vi "Subgroup Spectrum Lines.vi"(0 "spectra":T2(array[cluster]), 9 "system info in":refnum<class "EP System Info.lvclass">, 11 "error in (no error)":errorcluster) -> (4 "harmonic subgroups complex spectra":cluster{"f0":dbl, "df":dbl, "vectors":cdb[]}[](array[cluster]), 6 "interharmonic subgroups complex spectra":cluster{"f0":dbl, "df":dbl, "vectors":cdb[]}[](array[cluster]), 10 "system info out":refnum<class "EP System Info.lvclass">, 15 "error out":errorcluster)   [LabVIEW 2014, in "NI_EP_Power Quality.lvlib"]
doc: "Performs subgrouping of 10/12-cycle step spectra to harmonic and interharmonic spectra according to IEC 61000-4-7:2009. Use the Complex To Polar function to convert the results of this VI to magnitude and phase spectra. Use the Complex To Re/Im function to convert the results of this VI to real and imaginary spectra.\n\nThis VI supports measuring single-line and multiple-line systems."
uses:
  <vilib>/addons/Electrical Power/PQ/NI_EP_Power Quality.lvlib
  <vilib>/addons/Electrical Power/PQ/Common/Controls/ep_AI Data Channel.ctl
  <vilib>/addons/Electrical Power/PQ/Common/Classes/System Info/EP System Info.lvclass
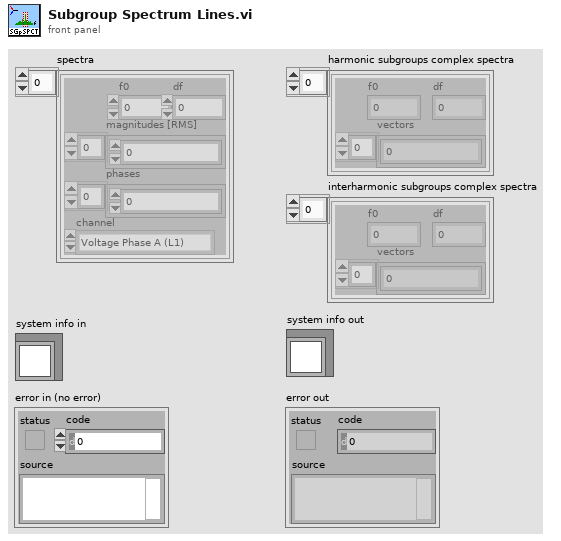
[diagram p1: front panel]
types:
  T1 = typedef "NI_EP_Power Quality.lvlib/ep_AI Data Channel.ctl" = enum16{"Voltage Phase A (L1)", "Voltage Phase B (L2)", "Voltage Phase C (L3)", "Voltage Phase N (Neutral)", "Current Phase A (L1)", "Current Phase B (L2)", "Current Phase C (L3)", "Current Phase N (Neutral)"}
  T2 = cluster{"f0":dbl, "df":dbl, "magnitudes [RMS]":dbl[], "phases":dbl[], "channel":T1}[]
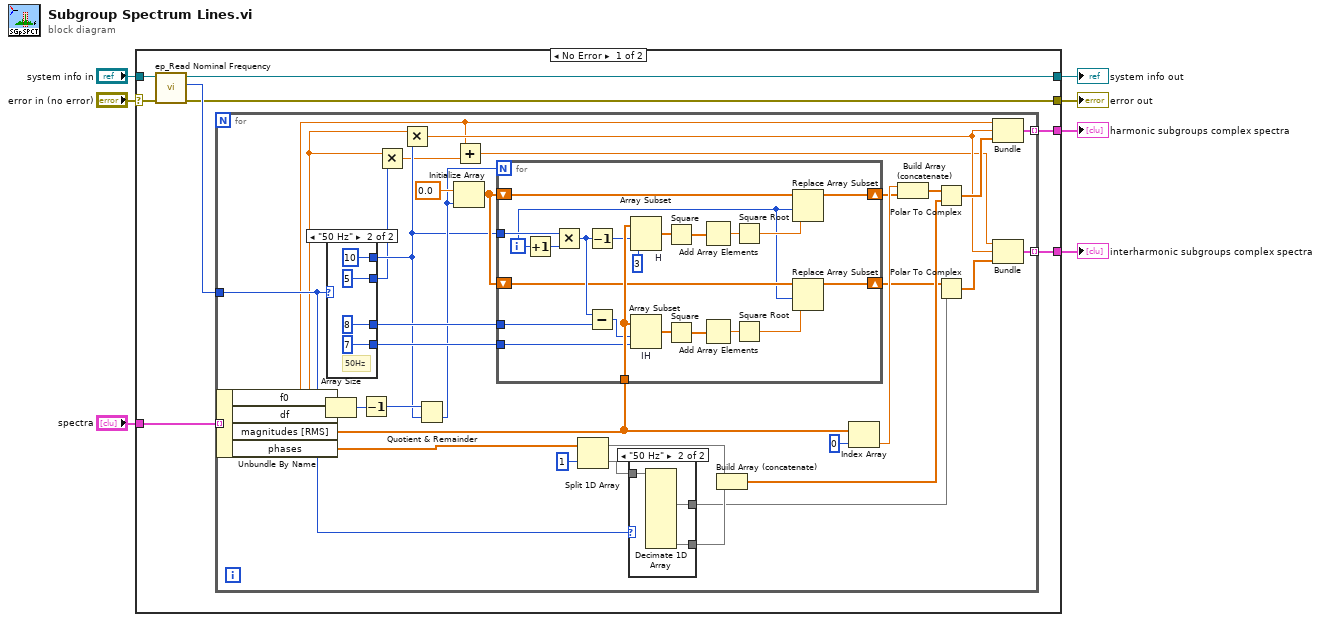
[diagram p0: block diagram]
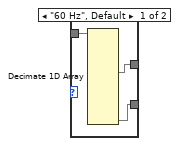
[diagram p2: hidden frame]
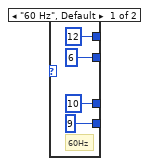
[diagram p3: hidden frame]
diagram:
  n1 = case shown="No Error" "error in (no error)" {
    selector: "error in (no error)" -> [w14 w86]
    tunnel: [w13 w86] -> w2
    tunnel: "system info in" -> [w12 w85]
    tunnel: [w11 w85] -> w4
    tunnel: "spectra" -> [w10 _]
    tunnel: [w9 _] -> w3
    tunnel: [w8 _] -> w1
    frame No Error {
      n2 = call <vilib>:"ep_Read Nominal Frequency.vi"("error in (no error)"=w14, "system info in"=w12) -> ("error out"=w13:errorcluster, "nominal frequency"=w15:enum16{"50 Hz", "60 Hz"}, "system info out"=w11:refnum<class "EP System Info.lvclass">)  [unwired: 6 in, 1 out]
      n3 = for {
        tunnel: w15 -> [w40]
        tunnel: w10 -> [w44] mode=indexing
        tunnel: [w43] -> w9 mode=indexing
        tunnel: [w16] -> w8 mode=indexing
        n4 = Unbundle By Name(w44) -> ("f0"=w18:dbl, "df"=w21:dbl, "magnitudes [RMS]"=w29:dbl[], "phases"=w30:dbl[])
        n5 = Array Size(array=w29) -> (size(s)=w32:i32)
        n6 = case shown="\"50 Hz\"" w40 {
          tunnel: [12 ("x") 10 ("x")] -> w26
          tunnel: [10 ("y") 8 ("y")] -> w46
          tunnel: [9 ("Array Length") 7 ("Array Length")] -> w45
          tunnel: [6 ("x") 5 ("x")] -> w20
          frame "60 Hz", Default {
            # "60Hz"
          }
          frame "50 Hz" {
            # "50Hz"
          }
        }
        n7 = Decrement(x=w32) -> (x-1=w31:i32)
        n8 = Multiply(x=w21, y=w20) -> (x*y=w19:dbl)
        n9 = Multiply(x=w21, y=w26) -> (x*y=w25:dbl)
        n10 = Quotient & Remainder(x=w31, y=w26) -> (floor(x/y)=w28:i32)  [unwired: 1 out]
        n11 = Initialize Array(0.0 ("Element Data"), w28) -> (w27:dbl[])
        n12 = Add(x=w18, y=w19) -> (x+y=w17:dbl)
        n13 = for {
          N: w28 -> [_]
          shift-right: [w68] -> w34
          shift-left: w27 -> [w84]
          tunnel: w29 -> [w83]
          tunnel: w26 -> [w80]
          tunnel: w46 -> [w82]
          tunnel: w45 -> [w81]
          shift-right: [w66] -> w24
          shift-left: w27 -> [w65]
          i -> [w63]
          n14 = Increment(x=w63) -> (x+1=w69:i32)
          n15 = Multiply(x=w80, y=w69) -> (x*y=w79:i32)
          n16 = Decrement(x=w79) -> (x-1=w75:i32)
          n17 = Subtract(x=w79, y=w82) -> (x-y=w76:i32)
          n18 = Array Subset "H"(array=w83, index=w75, length=3) -> (w78:dbl[])
          n19 = Array Subset "IH"(array=w83, index=w76, length=w81) -> (w77:dbl[])
          n20 = Square(x=w78) -> (x^2=w72:dbl[])
          n21 = Square(x=w77) -> (x^2=w73:dbl[])
          n22 = Add Array Elements(numeric array=w72) -> (sum=w71:dbl)
          n23 = Add Array Elements(numeric array=w73) -> (sum=w70:dbl)
          n24 = Square Root(x=w71) -> (sqrt(x)=w67:dbl)
          n25 = Square Root(x=w70) -> (sqrt(x)=w64:dbl)
          n26 = Replace Array Subset(array=w84, new element=w67, index=w63) -> (w68:dbl[])
          n27 = Replace Array Subset(array=w65, new element=w64, index=w63) -> (w66:dbl[])
        }
        n28 = Split 1D Array(array=w30, index=1) -> (first subarray=w36:dbl[], second subarray=w37:dbl[])
        n29 = case shown="\"50 Hz\"" w40 {
          tunnel: w37 -> [w51 w54]
          tunnel: [w50 w53] -> w39
          tunnel: [w49 w52] -> w23
          frame "60 Hz", Default {
            n30 = Decimate 1D Array(w51) -> (w49:dbl[], w50:dbl[])  [unwired: 10 out]
          }
          frame "50 Hz" {
            n31 = Decimate 1D Array(w54) -> (w52:dbl[], w53:dbl[])  [unwired: 8 out]
          }
        }
        n32 = Build Array (concatenate)(w36, w39) -> (w42:dbl[])
        n33 = Index Array(array=w29, index=0 ("Index")) -> (element=w35:dbl)
        n34 = Build Array (concatenate)(w35, w34) -> (w33:dbl[])
        n35 = Polar To Complex(1:w42, 2:w33) -> (0:w41:cdb[])
        n36 = Polar To Complex(1:w23, 2:w24) -> (0:w22:cdb[])
        n37 = Bundle("f0"=w18, w25, w41) -> (w43:cluster{"f0":dbl, dbl, cdb[]})  [unwired: 1 in]
        n38 = Bundle(w17, w25, w22) -> (w16:cluster{dbl, dbl, cdb[]})  [unwired: 1 in]
      }
    }
    frame Error {
    }
  }
  "error out" <- w2
  "harmonic subgroups complex spectra" <- w3
  "system info out" <- w4
  "interharmonic subgroups complex spectra" <- w1
